vi "Write engine.vi"(8 "error in (no error)":errorcluster, 10 "engine":string, 11 "Shared Memory Configuration in":refnum<class "Shared Memory Configuration.lvclass">) -> (0 "error out":errorcluster, 3 "Shared Memory Configuration out":refnum<class "Shared Memory Configuration.lvclass">)   [LabVIEW 2013, in "Shared Memory Configuration.lvclass"]
uses:
  Shared Memory Configuration.lvclass
  Shared Memory Configuration.lvclass/Shared Memory Configuration.ctl
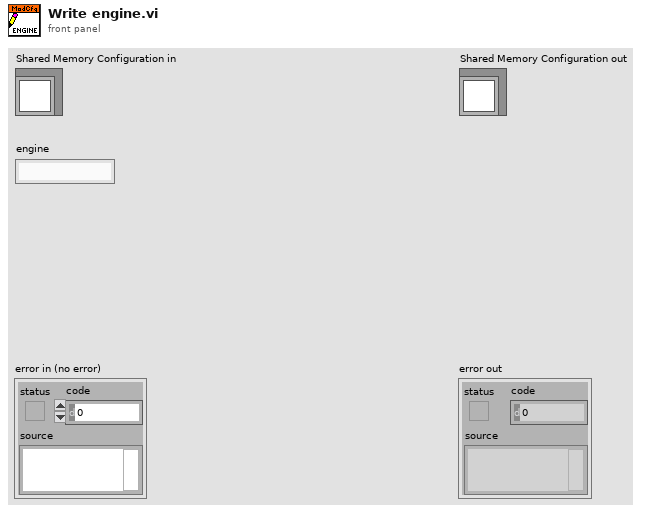
[diagram p1: front panel]
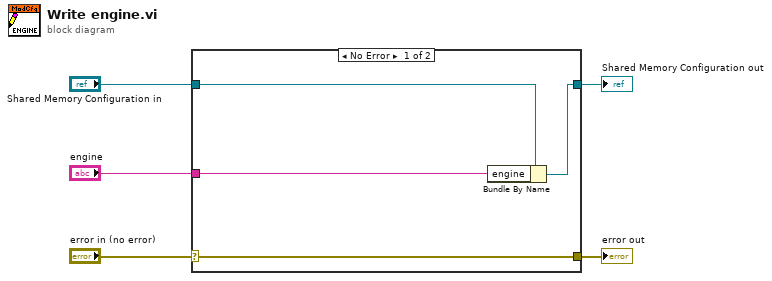
[diagram p0: block diagram]
diagram:
  n1 = case shown="No Error" "error in (no error)" {
    selector: "error in (no error)" -> [w9 w10]
    tunnel: [w9 w10] -> w4
    tunnel: [w7 w11] -> w2
    tunnel: "Shared Memory Configuration in" -> [w8 w11]
    tunnel: "engine" -> [w6 _]
    frame No Error {
      n2 = Bundle By Name(cluster=w8, "engine"=w6) -> (w7:refnum<class "Shared Memory Configuration.lvclass">)
    }
    frame Error {
    }
  }
  "error out" <- w4
  "Shared Memory Configuration out" <- w2
